vi "gui.vi"() -> ()   [LabVIEW 2020]
uses:
  <vilib>/Instr/_visa.llb/VISA Configure Serial Port (Instr).vi
panel:
  in  "stop":bool
  in  "VISA resource name 2":refnum<visa-resource-name>="COM5"
  in  "error in (no error) 2":errorcluster
  out "error out":errorcluster
  in  "Power (%)":dbl(slide)=100.0 scale=0.0..100.0
  in  "Shutter 2":bool
  out "Emitting:":bool=TRUE
  # "561 nm"
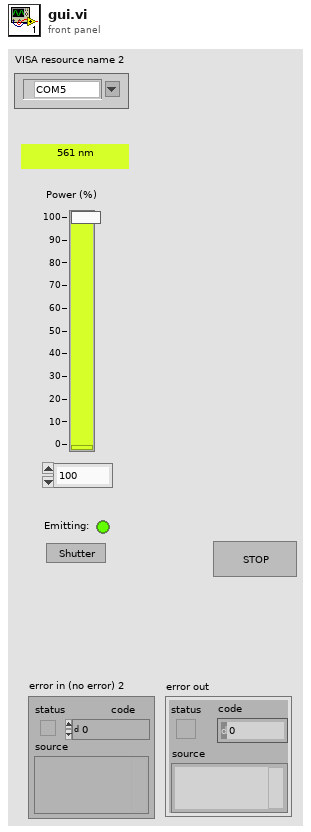
[diagram p1: front panel]
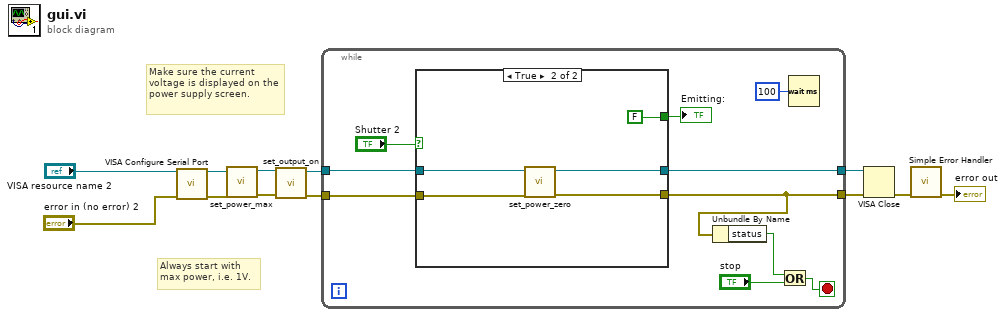
[diagram p0: block diagram]
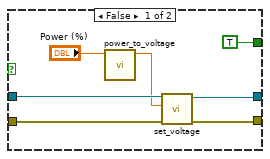
[diagram p2: hidden frame]
diagram:
  # "Make sure the current voltage is displayed on the power supply screen."
  # "Always start with\nmax power, i.e. 1V."
  n1 = call-poly "VISA Configure Serial Port"("VISA resource name"="VISA resource name 2", "error in (no error)"="error in (no error) 2") -> ("VISA resource name out"=w8:refnum<visa-resource-name>, "error out"=w7:errorcluster)  [unwired: 8 in, 4 out]
  n2 = call "set_power_max.vi"("error in 2"=w7, "VISA resource name 2"=w8) -> ("error out 2"=w3:errorcluster, "VISA resource name out"=w4:refnum<visa-resource-name>)  [unwired: 8 in]
  n3 = call "set_output_on.vi"("error in"=w3, "VISA resource name"=w4) -> ("error out"=w1:errorcluster, "VISA resource name out"=w2:refnum<visa-resource-name>)  [unwired: 8 in]
  n4 = while {
    tunnel: w2 -> [w22]
    tunnel: w1 -> [w21]
    tunnel: [w20] -> w5
    tunnel: [w19] -> w6
    stop <- w15 stop-if-true
    n5 = case shown="True" "Shutter 2" {
      tunnel: w22 -> [w28 w33]
      tunnel: w21 -> [w27 w31]
      tunnel: [w25 w30] -> w20
      tunnel: [w26 w32] -> w19
      tunnel: [TRUE ("Boolean") FALSE ("Boolean")] -> w17
      frame False {
        n6 = call "power_to_voltage.vi"("Power"="Power (%)") -> ("Voltage"=w23:dbl)  [unwired: 10 in]
        n7 = call "set_voltage.vi"("error in 2"=w27, "voltage"=w23, "VISA resource name 2"=w28) -> ("error out 2"=w25:errorcluster, "VISA resource name out"=w26:refnum<visa-resource-name>)  [unwired: 6 in, 1 out]
      }
      frame True {
        n8 = call "set_power_zero.vi"("error in 2"=w31, "VISA resource name 2"=w33) -> ("error out 2"=w30:errorcluster, "VISA resource name out"=w32:refnum<visa-resource-name>)  [unwired: 8 in]
      }
    }
    "Emitting:" <- w17
    n9 = Unbundle By Name(w20) -> ("status"=w14:bool)
    n10 = Or(x=w14, y="stop") -> (x .or. y?=w15:bool)
    n11 = Wait (ms)(milliseconds to wait=u32 100) -> ()  [unwired: 1 out]
  }
  n12 = VISA Close(VISA resource name=w6, error in (no error)=w5) -> (error out=w12:errorcluster)
  n13 = call <vilib>:"Simple Error Handler.vi"("error in (no error)"=w12) -> ("error out"=→"error out":errorcluster)  [unwired: 1 in, 7 out]
